vi "Send_simple_command.vi"(7 "index5 array":u8[](array[numeric]), 9 "Unit selection":u8, 10 "Unit port":u16, 11 "cmd #":u8) -> (3 "Cluster":T1)   [LabVIEW 2013]
uses:
  UDP_read_datagram.ctl
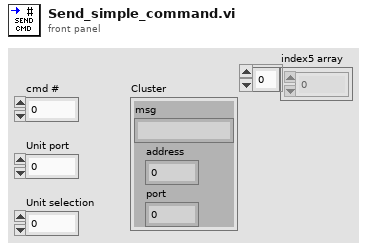
[diagram p1: front panel]
types:
  T1 = typedef "UDP_read_datagram.ctl" = cluster{"msg":string, "address":u32, "port":u16}
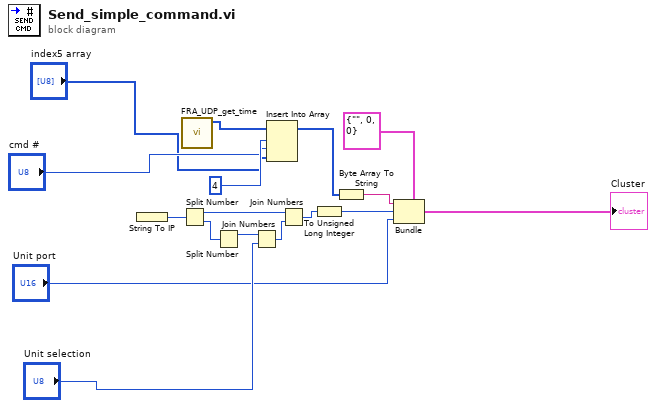
[diagram p0: block diagram]
diagram:
  n1 = String To IP() -> (0:w15:u32)  [unwired: 1 in]
  n2 = Split Number(x=w15) -> (hi(x)=w8:u16, lo(x)=w7:u16)
  n3 = call "FRA_UDP_get_time.vi"() -> ("array"=w13:u8[])  [unwired: 10 in, 1 out]
  n4 = Split Number(x=w7) -> (hi(x)=w10:u8)  [unwired: 1 out]
  n5 = Join Numbers(hi=w10, lo="Unit selection") -> ((hi.lo)=w9:u16)
  n6 = Insert Into Array(array=w13, index=4 ("new element/subarray"), new element #1="cmd #", new element #2="index5 array") -> (w14:u8[])
  n7 = Join Numbers(hi=w8, lo=w9) -> ((hi.lo)=w11:u32)
  n8 = To Unsigned Long Integer(number=w11) -> (unsigned 32bit integer=w12:u32)
  n9 = Byte Array To String(unsigned byte array=w14) -> (string=w6:string)
  n10 = Bundle(cluster=T1 {"msg"="", "address"=0, "port"=0}, "msg"=w6, "address"=w12, "port"="Unit port") -> (→"Cluster":T1)
